vi "Paralle.vi"() -> ()   [LabVIEW 2017]
panel:
  out "error out":errorcluster
  out "element":string
  in  "stop":bool
  in  "Array":string[](array[string])=["192.168.10.21", "192.168.10.23"]
  in  "error in (no error)":errorcluster
  in  "timeout (ms)":i32=10000
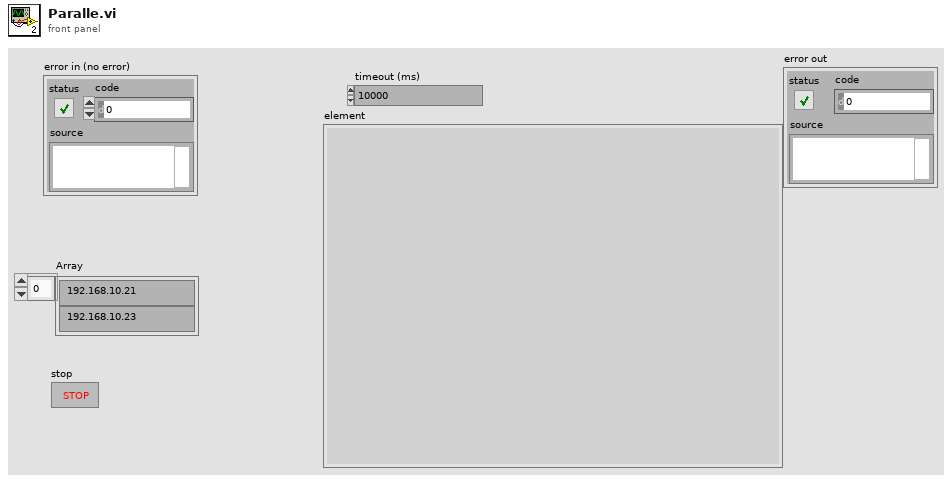
[diagram p1: front panel]
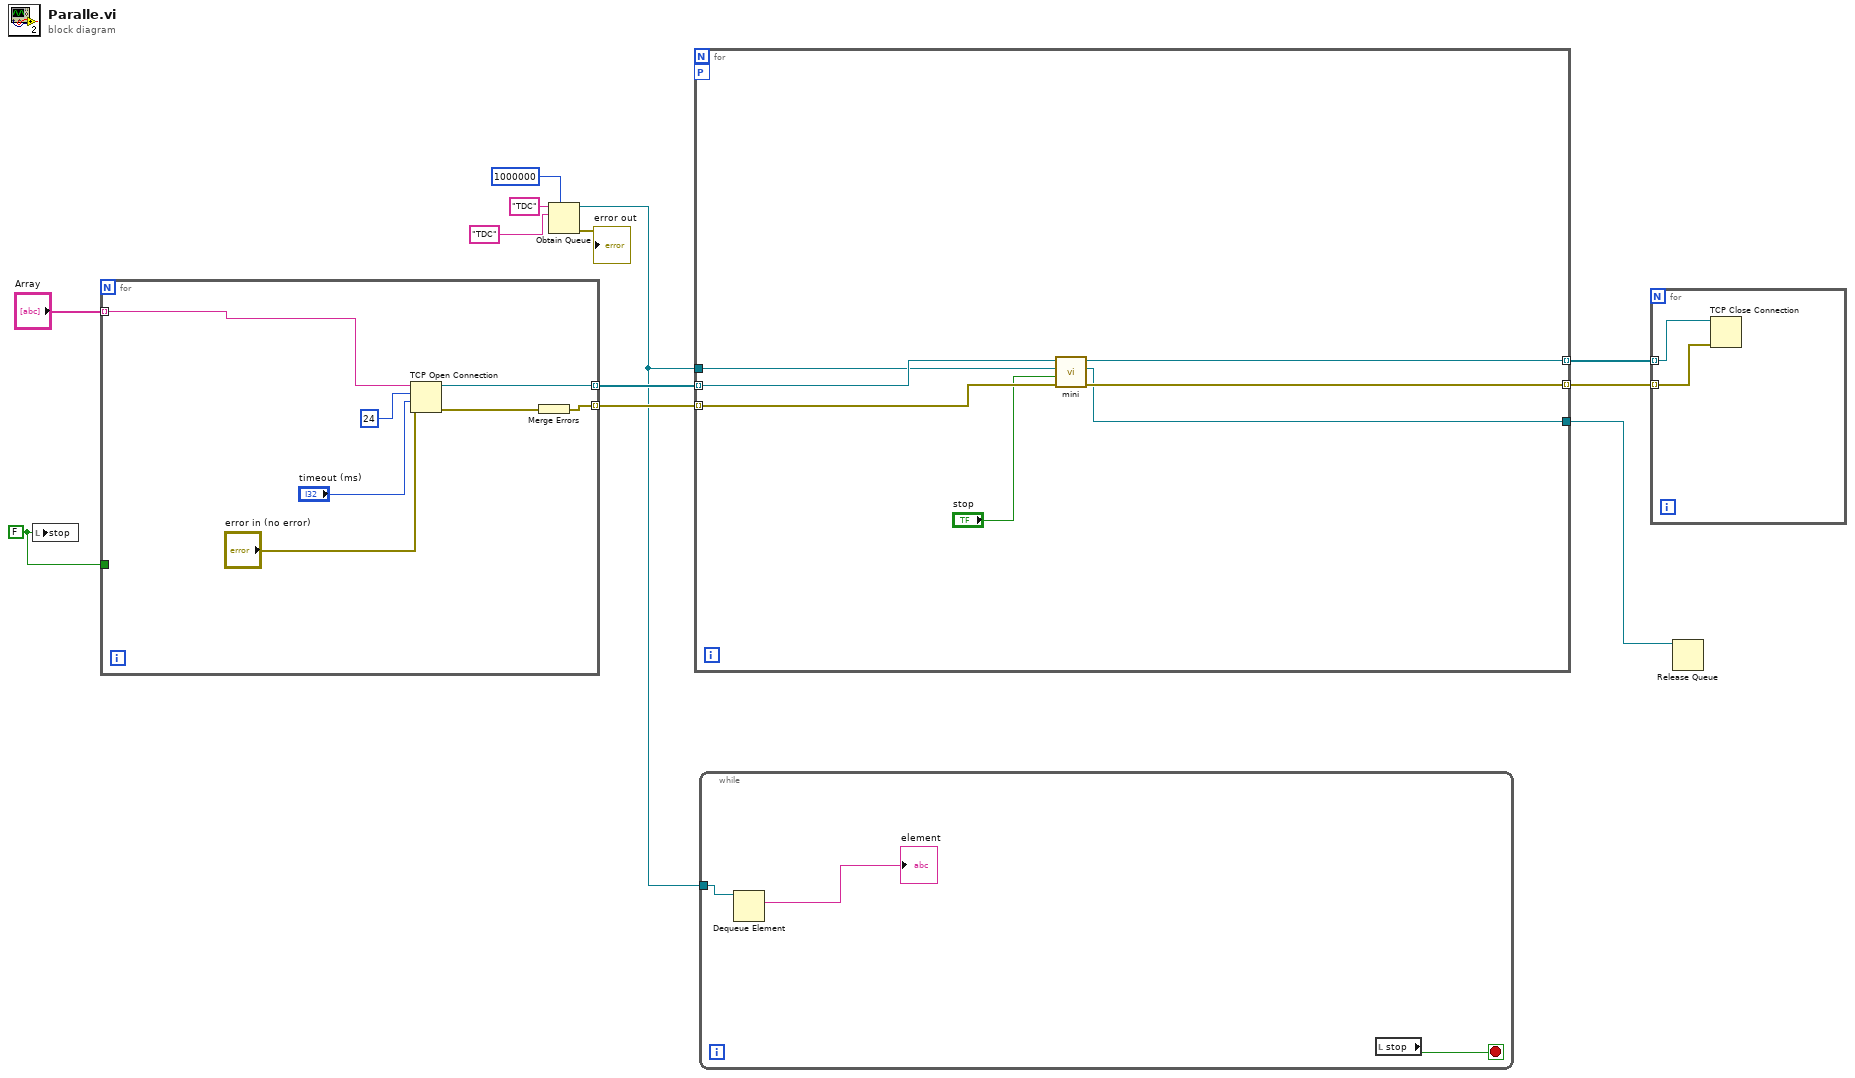
[diagram p0: block diagram]
diagram:
  w1 = FALSE ("stop")
  n1 = local write "stop"(w1) -> ()
  n2 = for {
    tunnel: "Array" -> [w16] mode=indexing
    tunnel: [w15] -> w11 mode=indexing
    tunnel: [w13] -> w10 mode=indexing
    tunnel: w1 -> [_]
    n3 = TCP Open Connection(address=w16, remote port or service name=u16 24 ("port"), timeout ms (60000)="timeout (ms)", error in (no error)="error in (no error)") -> (connection ID=w15:refnum<k5>, error out=w14:errorcluster)  [unwired: 1 in]
    n4 = Merge Errors(w14) -> (w13:errorcluster)
  }
  n5 = Obtain Queue(max queue size (-1, unlimited)=1000000, name (unnamed)="TDC", element data type="TDC" ("name (unnamed)")) -> (queue out=w4:refnum<queue>, error out=→"error out":errorcluster)  [unwired: 2 in, 1 out]
  n6 = for {
    tunnel: w11 -> [w26] mode=indexing
    tunnel: w10 -> [w25] mode=indexing
    tunnel: [w24] -> w9 mode=indexing
    tunnel: [w23] -> w8 mode=indexing
    workers-P: _ -> [_]
    tunnel: w4 -> [w21]
    tunnel: [w20] -> w2
    n7 = call "mini.vi"("error in (no error)"=w25, "stop"="stop", "queue out 2"=w21, "connection ID 2"=w26) -> ("error out 3"=w23:errorcluster, "queue out"=w20:refnum<queue>, "connection ID"=w24:refnum<k5>)  [unwired: 5 in]
  }
  n8 = while {
    tunnel: w4 -> [w27]
    stop <- w28 stop-if-true
    n9 = Dequeue Element(queue=w27) -> (element=→"element":string)  [unwired: 2 in, 3 out]
    n10 = local read "stop"() -> (w28:bool)
  }
  n11 = for {
    tunnel: w9 -> [w31] mode=indexing
    tunnel: w8 -> [w30] mode=indexing
    n12 = TCP Close Connection(connection ID=w31, error in (no error)=w30) -> ()  [unwired: 1 in, 2 out]
  }
  n13 = Release Queue(queue=w2) -> ()  [unwired: 2 in, 3 out]
